vi "NameCode.vi"(4 "# Z":i32, 5 "Name0":string="RAW-2048-", 6 "# BRtn extra":i32, 7 "# ARpt extra":i32=5, 8 "# B rpt":i32=1, 9 "# B scan":i32, 10 "# A rpt":i32, 11 "# Aline":i32) -> (1 "Scan Parameter":string, 2 "Name Code":string)   [LabVIEW 2017]
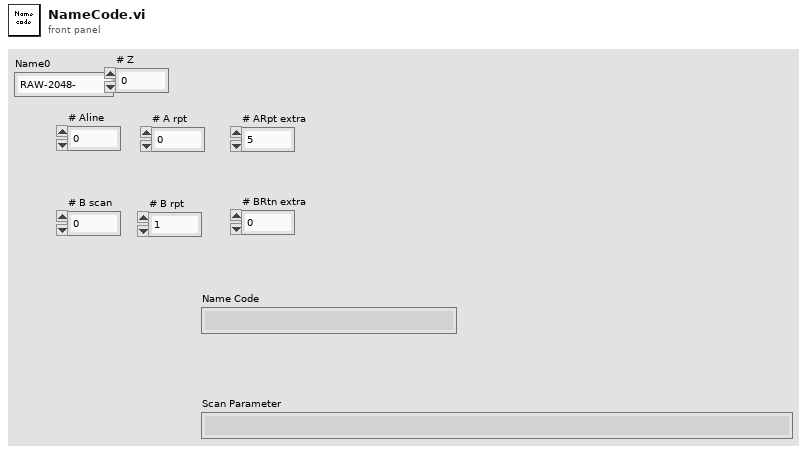
[diagram p1: front panel]
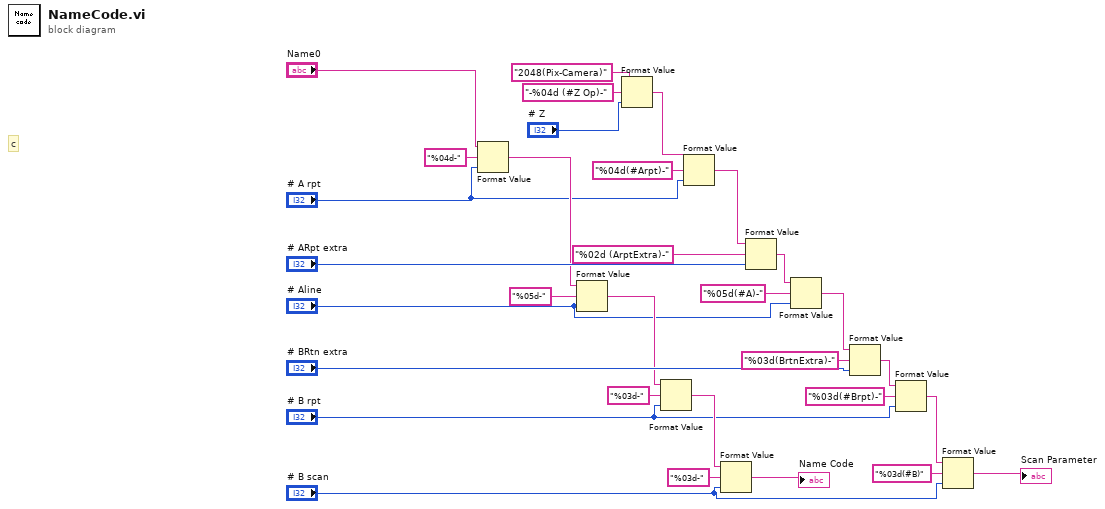
[diagram p0: block diagram]
diagram:
  # "c"
  n1 = Format Value(string ("")="Name0", format string="%04d-", value (0)="# A rpt") -> (output string=w19:string)
  n2 = Format Value(string ("")=w19, format string="%05d-", value (0)="# Aline") -> (output string=w18:string)
  n3 = Format Value(string ("")="2048(Pix-Camera)", format string="-%04d (#Z Op)-", value (0)="# Z") -> (output string=w15:string)
  n4 = Format Value(string ("")=w18, format string="%03d-", value (0)="# B rpt") -> (output string=w27:string)
  n5 = Format Value(string ("")=w15, format string="%04d(#Arpt)-", value (0)="# A rpt") -> (output string=w13:string)
  n6 = Format Value(string ("")=w27, format string="%03d-", value (0)="# B scan") -> (output string=→"Name Code":string)
  n7 = Format Value(string ("")=w13, format string="%02d (ArptExtra)-", value (0)="# ARpt extra") -> (output string=w11:string)
  n8 = Format Value(string ("")=w11, format string="%05d(#A)-", value (0)="# Aline") -> (output string=w9:string)
  n9 = Format Value(string ("")=w9, format string="%03d(BrtnExtra)-", value (0)="# BRtn extra") -> (output string=w7:string)
  n10 = Format Value(string ("")=w7, format string="%03d(#Brpt)-", value (0)="# B rpt") -> (output string=w3:string)
  n11 = Format Value(string ("")=w3, format string="%03d(#B)", value (0)="# B scan") -> (output string=→"Scan Parameter":string)
